vi "analyseImage.vi"(8 "error in (no error)":errorcluster, 10 "Array":T1(array[cluster]), 11 "AbsorptionAnalyser in":refnum<class "AbsorptionAnalyser.lvclass">) -> (0 "error out":errorcluster, 3 "AbsorptionAnalyser out":refnum<class "AbsorptionAnalyser.lvclass">)   [LabVIEW 2009, in "Tools.lvlib" / "Imaging.lvlib" / "AbsorptionAnalyser.lvclass"]
uses:
  AbsorptionAnalyser.lvclass
  Filing/FileNeologist/FileNeologist.lvclass
  ImageAnalyser.lvclass
  Filing/FileSystem/FileSystem.lvclass
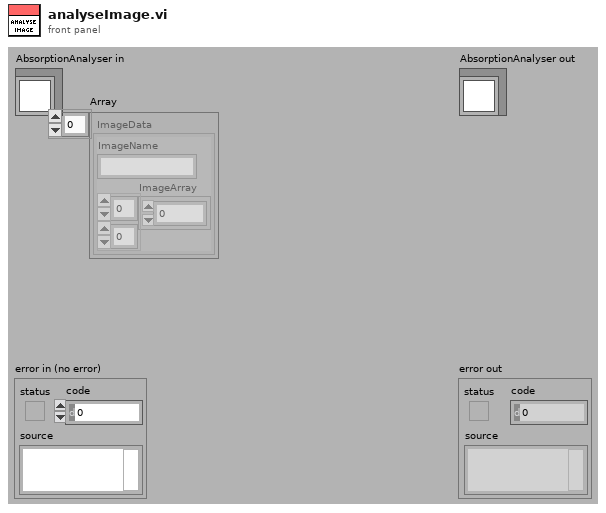
[diagram p1: front panel]
types:
  T1 = cluster{"ImageName":string, "ImageArray":sgl[][]}[]
  T2 = cluster{"Name":string, "Results":dbl[], "AnalysisType":string}
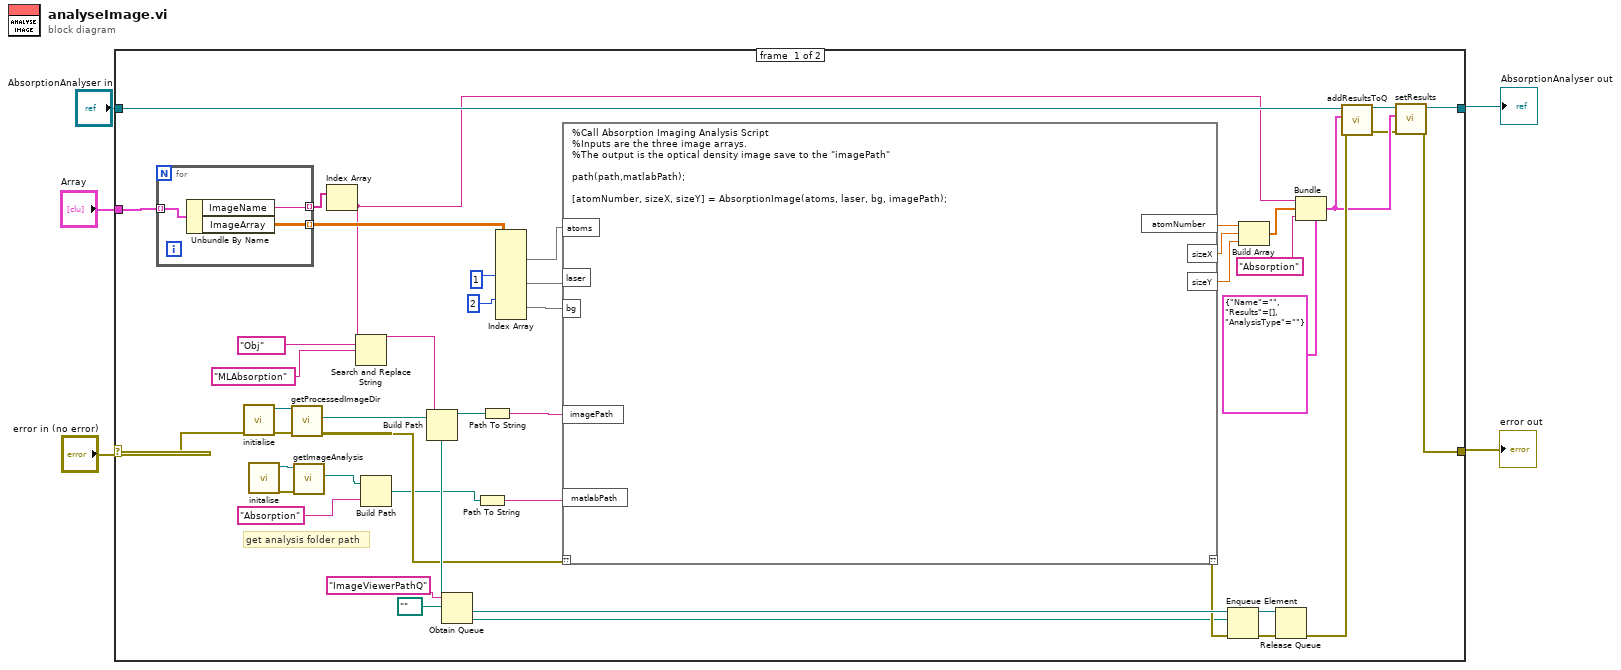
[diagram p0: block diagram]
diagram:
  n1 = case shown="No Error" "error in (no error)" {
    selector: "error in (no error)" -> [w18 w54]
    tunnel: [w6 w54] -> w4
    tunnel: [w9 w53] -> w2
    tunnel: "AbsorptionAnalyser in" -> [w48 w53]
    tunnel: "Array" -> [w47 _]
    frame #0 {
      # "get analysis folder path"
      n2 = for {
        tunnel: w47 -> [w52] mode=indexing
        tunnel: [w51] -> w46 mode=indexing
        tunnel: [w50] -> w41 mode=indexing
        n3 = Unbundle By Name(w52) -> ("ImageName"=w50:string, "ImageArray"=w51:sgl[][])
      }
      n4 = call "initialise.vi"("error in (no error)"=w18) -> ("error out"=w37:errorcluster, "FileNeologist out"=w38:refnum<class "FileNeologist.lvclass">)  [unwired: 9 in]
      n5 = call "initalise.vi"() -> ("error out"=w14:errorcluster, "FileSystem out"=w15:refnum<class "FileSystem.lvclass">)  [unwired: 10 in]
      n6 = call-dynamic "getProcessedImageDir.vi"("error in (no error)"=w37, "FileNeologist in"=w38) -> ("error out"=w17:errorcluster, "Path"=w36:path)  [unwired: 7 in, 1 out]
      n7 = call "getImageAnalysis.vi"("error in (no error)"=w14, "FileSystem in"=w15) -> ("ImageAnalysis"=w13:path)  [unwired: 7 in, 2 out]
      n8 = Index Array(array=w41) -> (element=w21:string)  [unwired: 1 in]
      n9 = Search and Replace String(input string=w21, search string="Obj", replace string="MLAbsorption") -> (result string=w35:string)  [unwired: 5 in, 3 out]
      n10 = Build Path(base path=w13, name or relative path="Absorption") -> (appended path=w11:path)
      n11 = Build Path(base path=w36, name or relative path=w35) -> (appended path=w24:path)
      n12 = Obtain Queue(name (unnamed)="ImageViewerPathQ", element data type=path "") -> (queue out=w32:refnum<queue>)  [unwired: 3 in, 2 out]
      n13 = Path To String(path=w11) -> (string=w16:string)
      n14 = Path To String(path=w24) -> (string=w29:string)
      n15 = Index Array(array=w46, index (dim 0) #2=1, index (dim 0) #3=2) -> (element #1=w44:sgl[][], element #2=w43:sgl[][], element #3=w42:sgl[][])  [unwired: 7 in]
      n16 = script code="%Call Absorption Imaging Analysis Script \n%Inputs are the three image arrays.\n%The output is the optical density image save to the \"imagePath\"\n\npath(path,matlabPath);\n\n[atomNumber, sizeX, sizeY] = AbsorptionImage(atoms, laser, bg, imagePath);"("??"=w17, "bg"=w42, "laser"=w43, "atoms"=w44, "imagePath"=w29, "matlabPath"=w16) -> ("??"=w25:errorcluster, "atomNumber"=w28:dbl, "sizeX"=w27:dbl, "sizeY"=w26:dbl)
      n17 = Enqueue Element(queue=w32, element=w24, error in (no error)=w25) -> (queue out=w31:refnum<queue>, error out=w30:errorcluster)  [unwired: 1 in, 1 out]
      n18 = Build Array(w28, w27, w26) -> (w22:dbl[])
      n19 = Release Queue(queue=w31, error in (no error)=w30) -> (error out=w23:errorcluster)  [unwired: 1 in, 2 out]
      n20 = Bundle(cluster=T2 {"Name"="", "Results"=[], "AnalysisType"=""} ("output cluster"), "Name"=w21, "Results"=w22, "AnalysisType"="Absorption") -> (w8:T2)
      n21 = call "addResultsToQ.vi"("error in (no error)"=w23, "Results"=w8, "ImageAnalyser in"=w48) -> ("error out"=w7:errorcluster, "ImageAnalyser out"=w10:refnum<class "AbsorptionAnalyser.lvclass">)  [unwired: 7 in]
      n22 = call "setResults.vi"("error in (no error)"=w7, "results"=w8, "ImageAnalyser in"=w10) -> ("error out"=w6:errorcluster, "ImageAnalyser out"=w9:refnum<class "AbsorptionAnalyser.lvclass">)  [unwired: 7 in]
    }
    frame #1 {
    }
  }
  "error out" <- w4
  "AbsorptionAnalyser out" <- w2
